vi "MatrixReset.vi"(8 "error in (no error)":errorcluster, 11 "LXIPXISwitching in":refnum<class "LXIPXISwitching.lvclass">) -> (0 "error out":errorcluster, 3 "LXIPXISwitching out":refnum<class "LXIPXISwitching.lvclass">)   [LabVIEW 2018, in "LXIPXISwitching.lvclass"]
uses:
  LXIPXISwitching.lvclass
  LXIPXISwitching.lvclass/LXIPXISwitching.ctl
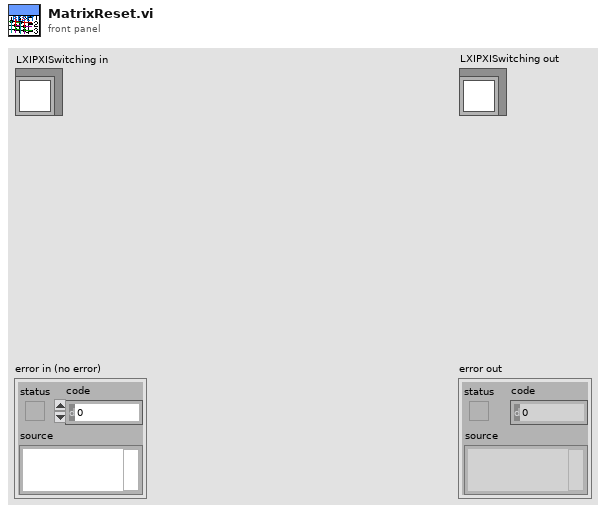
[diagram p1: front panel]
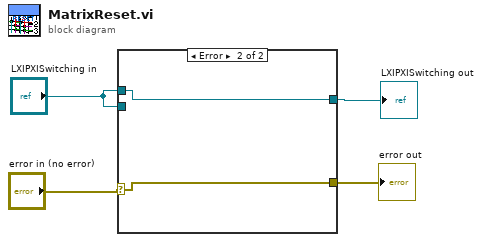
[diagram p0: block diagram]
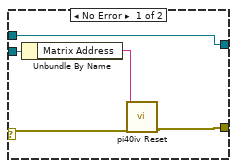
[diagram p2: hidden frame]
diagram:
  n1 = case shown="Error" "error in (no error)" {
    selector: "error in (no error)" -> [w7 w10]
    tunnel: [w8 w10] -> w1
    tunnel: [w6 w11] -> w2
    tunnel: "LXIPXISwitching in" -> [w6 w11]
    tunnel: "LXIPXISwitching in" -> [w5 _]
    frame No Error {
      n2 = Unbundle By Name(w5) -> ("Matrix Address"=w9:string)
      n3 = call <instrlib>:"pi40iv Reset.vi"("error in (no error)"=w7, "instrument handle"=w9) -> ("error out"=w8:errorcluster)  [unwired: 8 in, 1 out]
    }
    frame Error {
    }
  }
  "error out" <- w1
  "LXIPXISwitching out" <- w2
